vi "main_PosProcessamento_UDP_NI.vi"() -> ()   [LabVIEW 2019]
panel:
  out "Numeric 2":i32
  out "Numeric":i32
  in  "pos_processar 2":string
  in  "stop":bool
  in  "process_one":bool
  in  "process_all":bool
  out "filenames":string[](array[string])
  # "/"
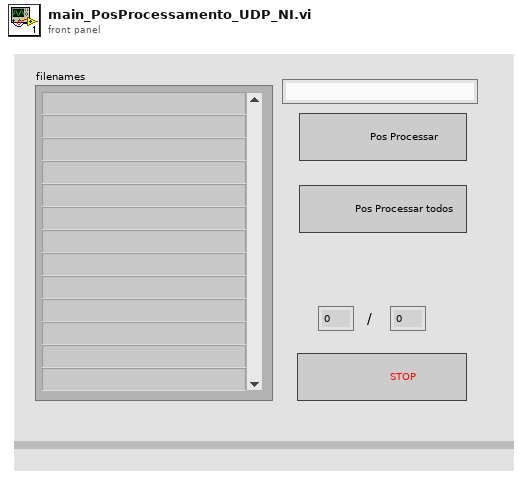
[diagram p1: front panel]
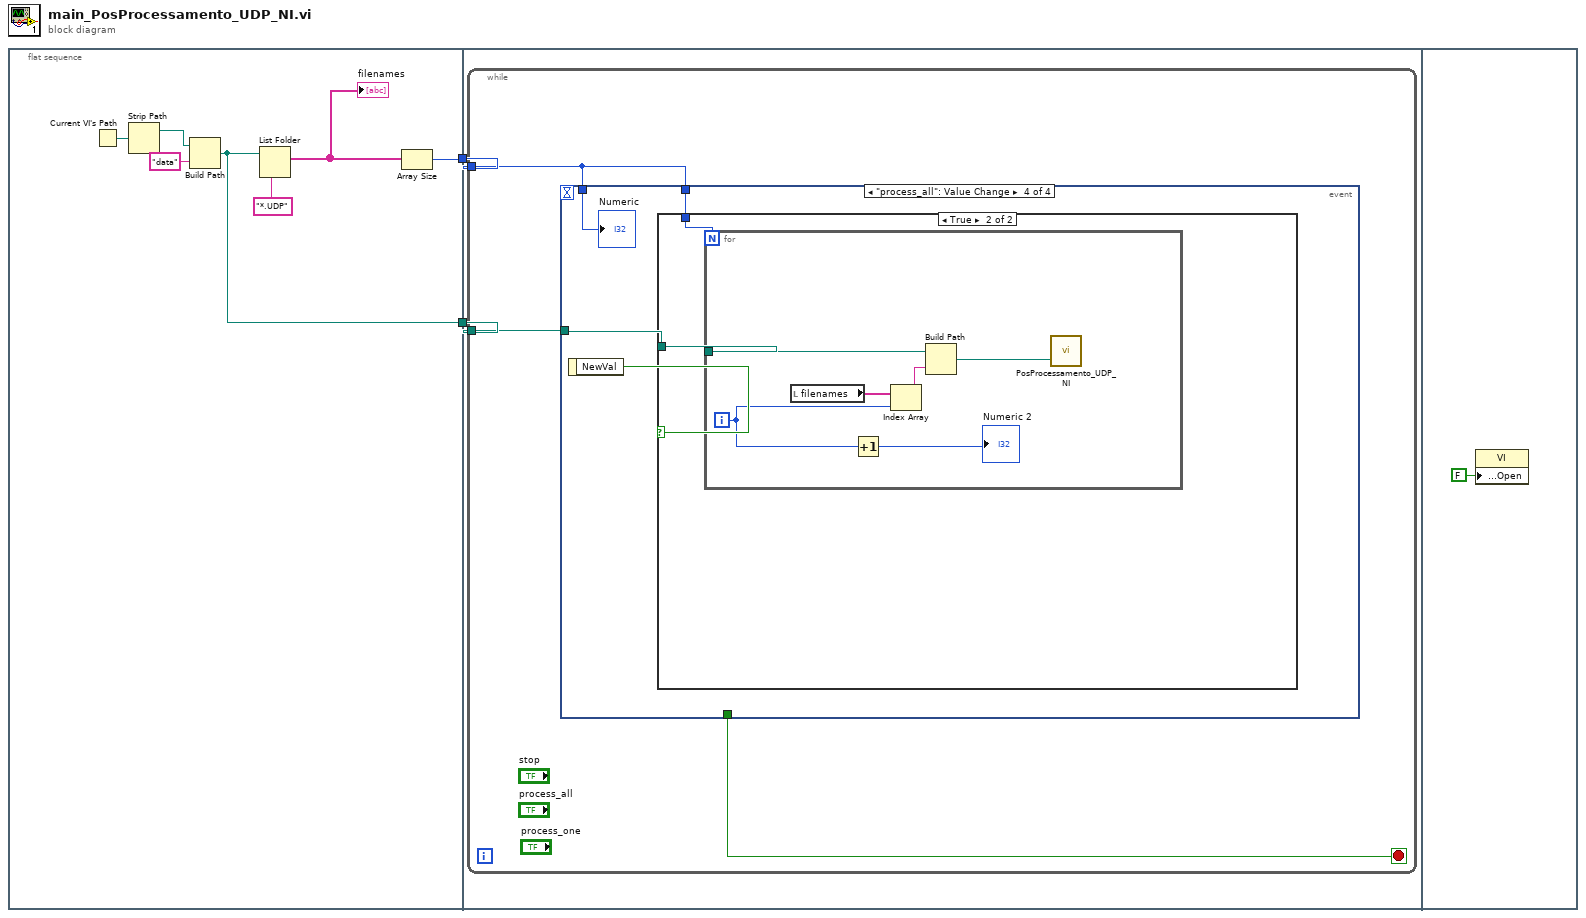
[diagram p0: block diagram]
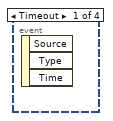
[diagram p2: hidden frame]
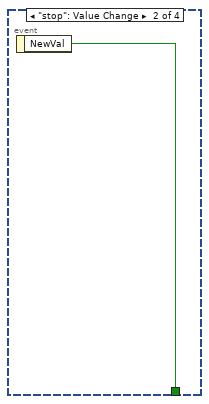
[diagram p3: hidden frame]
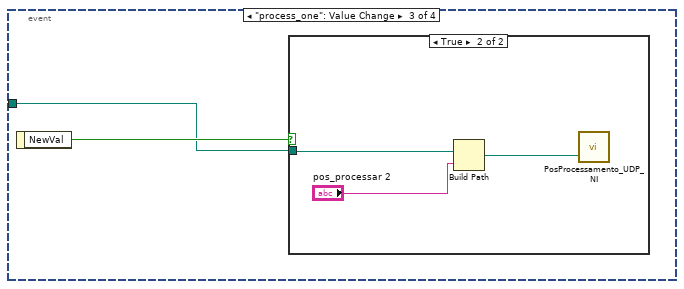
[diagram p4: hidden frame]
diagram:
  n1 = flat-sequence {
    tunnel: [w4] -> w2
    tunnel: [w3] -> w1
    tunnel: w2 -> [w11]
    tunnel: w1 -> [w10]
    frame #0 {
      n2 = Current VI's Path() -> (path=w8:path)
      n3 = Strip Path(path=w8) -> (stripped path=w7:path)  [unwired: 1 out]
      n4 = Build Path(base path=w7, name or relative path="data") -> (appended path=w3:path)
      n5 = List Folder(path=w3, pattern="*.UDP") -> (filenames=w5:string[])  [unwired: 2 in, 3 out]
      "filenames" <- w5
      n6 = Array Size(array=w5) -> (size(s)=w4:i32)
    }
    frame #1 {
      n7 = while {
        tunnel: w11 -> [w12]
        tunnel: w10 -> [w14]
        stop <- w13 stop-if-true
        n8 = event shown="[3] \"process_all\": Value Change" {
          selector: _ -> [_ _ _ _]
          dyn-events: _ -> [_ _ _ _]
          timeout: _ -> [_ _ _ _]
          tunnel: w14 -> [_ _ w16 w23]
          tunnel: w12 -> [_ _ _ w22]
          tunnel: [_ w15 _ _] -> w13
          tunnel: w12 -> [_ _ _ w21]
          event Timeout {
            n9 = event-data() -> ()  [unwired: 1 in, 3 out]
          }
          event "stop": Value Change {
            n10 = event-data() -> ("NewVal"=w15:bool)  [unwired: 1 in]
          }
          event "process_one": Value Change {
            n11 = event-data() -> ("NewVal"=w17:bool)  [unwired: 1 in]
            n12 = case shown="True" w17 {
              tunnel: w16 -> [_ w18]
              frame False {
              }
              frame True {
                n13 = Build Path(base path=w18, name or relative path="pos_processar 2") -> (appended path=w19:path)
                n14 = call "PosProcessamento_UDP_NI.vi"("file path (dialog if empty)"=w19) -> ()  [unwired: 2 in]
              }
            }
          }
          event "process_all": Value Change {
            n15 = event-data() -> ("NewVal"=w24:bool)  [unwired: 1 in]
            n16 = case shown="True" w24 {
              tunnel: w23 -> [_ w26]
              tunnel: w22 -> [_ w25]
              frame False {
              }
              frame True {
                n17 = for {
                  N: w25 -> [_]
                  tunnel: w26 -> [w29]
                  i -> [w28]
                  n18 = local read "filenames"() -> (w32:string[])
                  n19 = Increment(x=w28) -> (x+1=→"Numeric 2":i32)
                  n20 = Index Array(array=w32, index=w28) -> (element=w31:string)
                  n21 = Build Path(base path=w29, name or relative path=w31) -> (appended path=w30:path)
                  n22 = call "PosProcessamento_UDP_NI.vi"("file path (dialog if empty)"=w30) -> ()  [unwired: 2 in]
                }
              }
            }
            "Numeric" <- w21
          }
        }
      }
    }
    frame #2 {
      n23 = property class="VI"("Front Panel.Open"=FALSE ("Front Panel Window:Open")) -> ()  [unwired: 2 in, 2 out]
    }
  }
